vi "Mixed type array experiment JDP.vi"() -> ()   [LabVIEW 2011]
doc: "Demonstrates the use of the Variant JSON VIs for converting to and from a complex cluster."
uses:
  JSON Value/Set from JSON string.vi
  JSON Value/Get as JSON string.vi
  JSON Object/Set Object Item by name.vi
  JSON Value/Get Array by name.vi
  JSON Array/Set JSON Array.vi
  Variant JSON/Get as Variant.vi
  Variant JSON/Variant to JSON.vi
  JSON Value/Get Item by name array.vi
  JSON Value/JSON Value.lvclass
  JSON Object/JSON Object.lvclass
  Get Polymorphic/JSON GetSet.lvlib
  Variant JSON/Variant JSON.lvlib
  JSON Array/JSON Array.lvclass
panel:
  out "Same result":bool
  out "rebuilt instruments array for saving 2":string
  out "instruments out":cluster{"type":string, "config":string}[](array[cluster])
  in  "Defined structure (Note the <JSON> tag)":cluster{"type":string, "<JSON>config":string}[](array[cluster])
  out "rebuilt instruments array for saving":string
  out "type":T1(array[ring])
  out "config":string[](array[string])
  in  "Application Config":string="{\"instruments\":[{\"type\":\"SimMultimeter\",\"config\":{\"maxV\":10,\"maxI\":5}},\n{\"type\":\"SimVoltmeter\",\"config\": {\"Voltage\":100}},\n{\"type\":\"SimDAQ\",\"config\": 12.3}],\n\"etc.\":\"...\"\n}"
  # "Experiments in using JSON to hold configurations for application subcomponents, where the application code does not depend on the exact structure of the config past to the subcomponents."
  # "1. This method works now:"
  # "2. This method works, but only by tagging some LVstrings as being JSON text, rather that text in a JSON string"
  # "Modification: allow a <JSON> tag starting string name to identify it as JSON in the Variant functions"
  # "[{\"type\":\"SimMultimeter\",\"config\":{\"maxV\":10,\"maxI\",5}},\n{\"type\":\"SimVoltmeter\",\"config\": {\"maxV\":100}},\n{\"type\":\"SimDAQ\",\"config\": NULL}]"
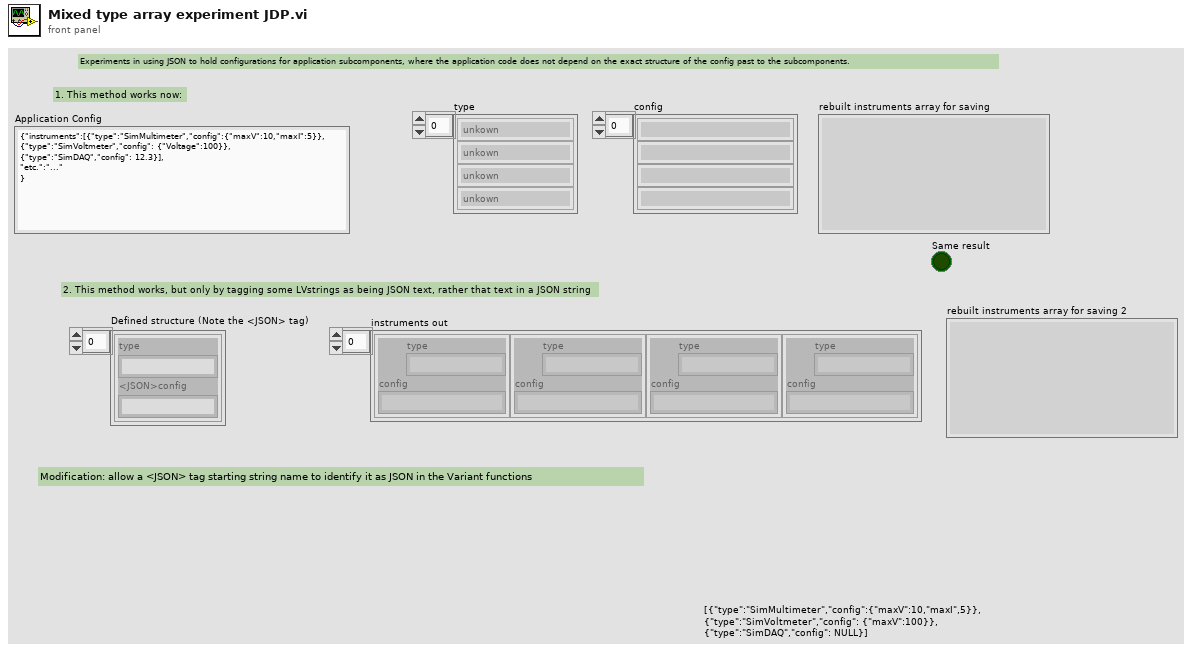
[diagram p1: front panel]
types:
  T1 = enum16{"unkown", "SimMultimeter", "SimDAQ", "SimVoltmeter"}[]
  T2 = enum16{"unkown", "SimMultimeter", "SimDAQ", "SimVoltmeter"}
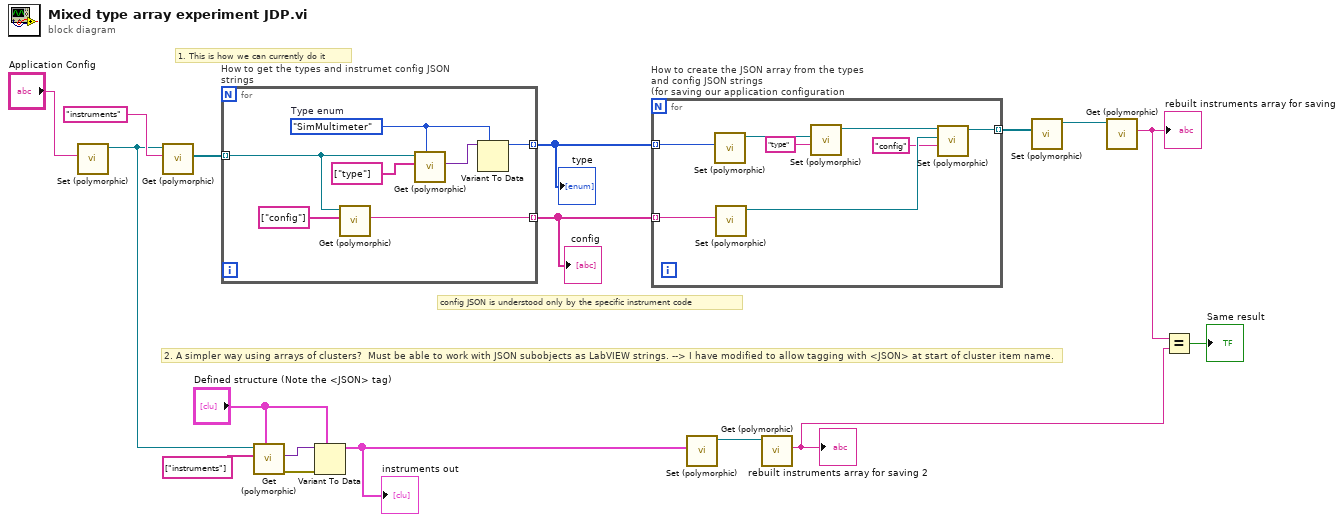
[diagram p0: block diagram]
diagram:
  # "1. This is how we can currently do it"
  # "2. A simpler way using arrays of clusters?  Must be able to work with JSON subobjects as LabVIEW strings. --> I have modified to allow tagging with <JSON> at start of cluster item name."
  # "config JSON is understood only by the specific instrument code"
  n1 = call-poly "Set (polymorphic).vi"("JSON stream"="Application Config") -> ("JSON Value out"=w10:refnum<class "JSON Value.lvclass">)  [unwired: 8 in, 2 out]
  n2 = call-poly "Get (polymorphic).vi"("name"="instruments", "JSON Value In"=w10) -> ("Array"=w16:refnum<class "JSON Value.lvclass">[])  [unwired: 6 in, 3 out]
  n3 = for "How to get the types and instrumet config JSON strings" {
    tunnel: w16 -> [w18] mode=indexing
    tunnel: [w23] -> w13 mode=indexing
    tunnel: [w20] -> w14 mode=indexing
    w19 = T2."SimMultimeter"  # Type enum
    n4 = call-poly "Get (polymorphic).vi"("Name Array"=string[] ["config"], "JSON Value in"=w18) -> ("String"=w23:string)  [unwired: 8 in, 1 out]
    n5 = call-poly "Get (polymorphic).vi"("Variant (Data Type)"=w19, "Name Array"=string[] ["type"], "JSON in"=w18) -> ("Variant out"=w21:variant)  [unwired: 6 in, 2 out]
    n6 = Variant To Data(type=w19, Variant=w21) -> (data=w20:T2)  [unwired: 1 in, 1 out]
  }
  "config" <- w13
  "type" <- w14
  n7 = call-poly "Get (polymorphic).vi"("Variant (Data Type)"="Defined structure (Note the <JSON> tag)", "Name Array"=string[] ["instruments"], "JSON in"=w10) -> ("error out"=w7:errorcluster, "Variant out"=w9:variant)  [unwired: 6 in, 1 out]
  n8 = Variant To Data(error in=w7, type="Defined structure (Note the <JSON> tag)", Variant=w9) -> (data=w5:cluster{"type":string, "<JSON>config":string}[])  [unwired: 1 out]
  "instruments out" <- w5
  n9 = for "How to create the JSON array from the types and config JSON strings\n(for saving our application configuration" {
    tunnel: w14 -> [w32] mode=indexing
    tunnel: w13 -> [w31] mode=indexing
    tunnel: [w25] -> w12 mode=indexing
    n10 = call-poly "Set (polymorphic).vi"("Variant"=w32) -> ("JSON Value out"=w30:refnum<class "JSON Value.lvclass">)  [unwired: 9 in, 1 out]
    n11 = call-poly "Set (polymorphic).vi"("JSON stream"=w31) -> ("JSON Value out"=w27:refnum<class "JSON Value.lvclass">)  [unwired: 8 in, 2 out]
    n12 = call-poly "Set (polymorphic).vi"("name"="type", "Value"=w30) -> ("JSON Object out"=w28:refnum<class "JSON Object.lvclass">)  [unwired: 7 in, 2 out]
    n13 = call-poly "Set (polymorphic).vi"("name"="config", "Value"=w27, "JSON Object in"=w28) -> ("JSON Object out"=w25:refnum<class "JSON Object.lvclass">)  [unwired: 6 in, 2 out]
  }
  n14 = call-poly "Set (polymorphic).vi"("Variant"=w5) -> ("JSON Value out"=w4:refnum<class "JSON Value.lvclass">)  [unwired: 9 in, 1 out]
  n15 = call-poly "Get (polymorphic).vi"("JSON Value in"=w4) -> ("String"=w2:string)  [unwired: 9 in, 1 out]
  "rebuilt instruments array for saving 2" <- w2
  n16 = call-poly "Set (polymorphic).vi"("Array"=w12) -> ("JSON Array out"=w11:refnum<class "JSON Array.lvclass">)  [unwired: 9 in, 1 out]
  n17 = call-poly "Get (polymorphic).vi"("JSON Value in"=w11) -> ("String"=w3:string)  [unwired: 9 in, 1 out]
  "rebuilt instruments array for saving" <- w3
  n18 = Equal?(x=w3, y=w2) -> (x = y?=→"Same result":bool)
